vi "TAT_PLC_Data_read_BOLLEAN_ALARM.vi"(7 "Enum":enum16{"Read", "Write"}(ring), 8 "error in (no error)":errorcluster, 10 "Array":bool[](array[boolean])) -> (0 "error out":errorcluster, 2 "Array 2":bool[](array[boolean]))   [LabVIEW 2017]
panel:
  # "STATION 1"
  # "ALARMS\t\nSR.NO\tPLC ALARMS\tDESCRIPTION\tTO SOFTWARE MEMORY BIT\n1\tM501\tEMERGENCY PRESSED\t8693\n2\tM502\tAIR PRESSURE NG\t8694\n3\tM503\tAUTO MODE NOT SELECT\t8695\n4\tM504\tMANUAL MODE NOT SELECT\t8696\n5\tM505\tSAFETY SENSOR NG\t8697\n6\tM506\tTOUCH BUTTON NG\t8698\n7\tM507\tPUSHER HOME RS NG\t8699\n8\tM508\tPUSHER END RS NG\t8700\n9\tM509\tTHREAD LOCKER CYL HOME RS NG\t8701\n10\tM510\tTHREAD LOCKER CYL END RS NG\t8702\n11\tM511\tPART CLAMP RS NG\t8703\n12\tM512\tDOOR 1 NG\t8704\n13\tM513\tDOOR 2 NG\t8705\n14\tM514\tHOLE BLOCK\t8706\n15\tM515\tSOFTWARE NOT RUN\t8707\n16\tM516\t\t8708\n17\tM517\t\t8709\n18\tM518\t\t8710"
  # "CONTROL PROCESS TO  LABVIEW from PLC"
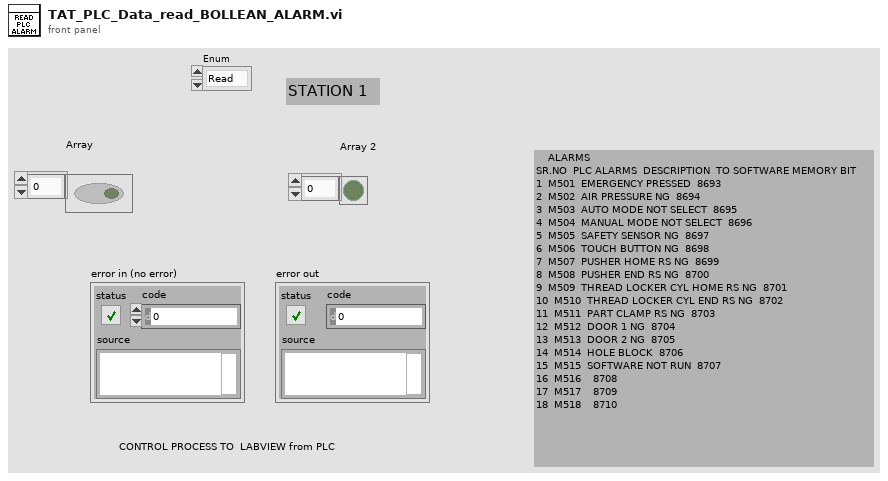
[diagram p1: front panel]
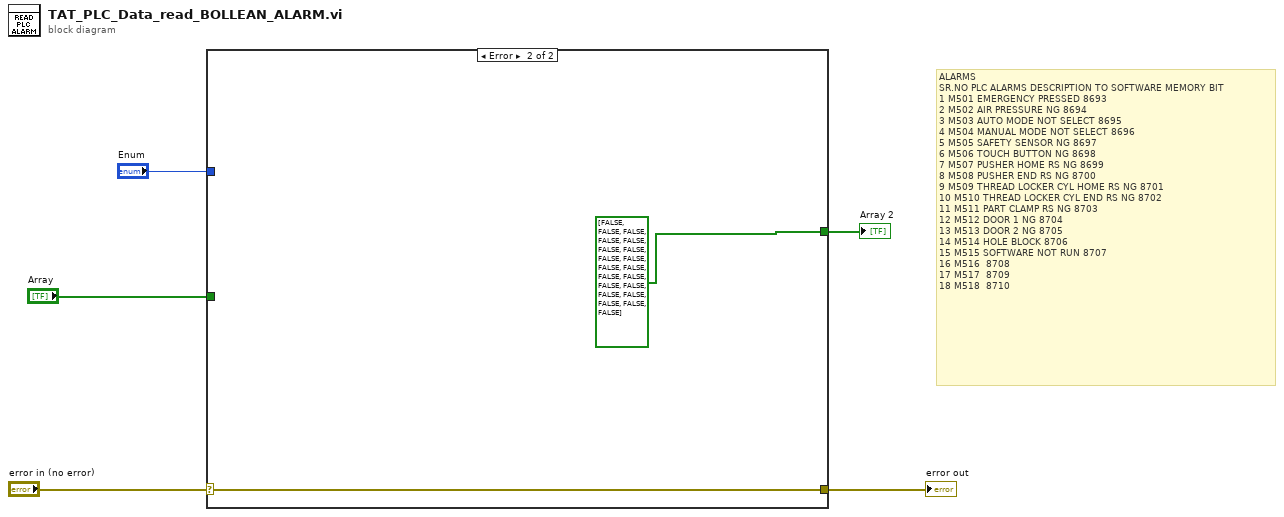
[diagram p0: block diagram]
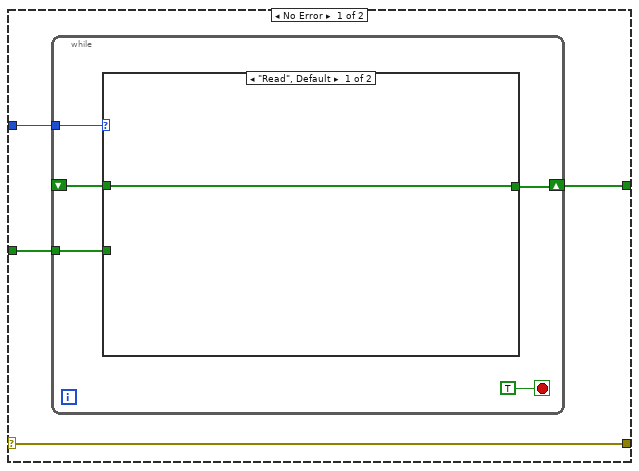
[diagram p2: hidden frame]
diagram:
  # "ALARMS\t\nSR.NO\tPLC ALARMS\tDESCRIPTION\tTO SOFTWARE MEMORY BIT\n1\tM501\tEMERGENCY PRESSED\t8693\n2\tM502\tAIR PRESSURE NG\t8694\n3\tM503\tAUTO MODE NOT SELECT\t8695\n4\tM504\tMANUAL MODE NOT SELECT\t8696\n5\tM505\tSAFETY SENSOR NG\t8697\n6\tM506\tTOUCH BUTTON NG\t8698\n7\tM507\tPUSHER HOME RS NG\t8699\n8\tM508\tPUSHER END RS NG\t8700\n9\tM509\tTHREAD LOCKER CYL HOME RS NG\t8701\n10\tM510\tTHREAD LOCKER CYL END RS NG\t8702\n11\tM511\tPART CLAMP RS NG\t8703\n12\tM512\tDOOR 1 NG\t8704\n13\tM513\tDOOR 2 NG\t8705\n14\tM514\tHOLE BLOCK\t8706\n15\tM515\tSOFTWARE NOT RUN\t8707\n16\tM516\t\t8708\n17\tM517\t\t8709\n18\tM518\t\t8710"
  n1 = case shown="Error" "error in (no error)" {
    selector: "error in (no error)" -> [w6 w18]
    tunnel: [w6 w18] -> w5
    tunnel: "Enum" -> [w9 _]
    tunnel: "Array" -> [w8 _]
    tunnel: [w7 bool[] [FALSE, FALSE, FALSE, FALSE, FALSE, FALSE, FALSE, FALSE, FALSE, FALSE, FALSE, FALSE, FALSE, FALSE, FALSE, FALSE, FALSE, FALSE, FALSE, FALSE]] -> w1
    frame No Error {
      n2 = while {
        tunnel: w9 -> [w13]
        shift-right: [w10] -> w7
        shift-left: _ -> [w11]
        tunnel: w8 -> [w12]
        stop <- TRUE stop-if-true
        n3 = case shown="\"Read\", Default" w13 {
          tunnel: w12 -> [_ w16]
          tunnel: [w15 w16] -> w10
          tunnel: w11 -> [w15 _]
          frame "Read", Default {
          }
          frame "Write" {
          }
        }
      }
    }
    frame Error {
    }
  }
  "error out" <- w5
  "Array 2" <- w1
